vi "update FPS slider.vi"(8 "error in (no error)":errorcluster, 11 "Thorcam in":refnum<class "Thorcam.lvclass">) -> (0 "error out":errorcluster, 3 "Thorcam out":refnum<class "Thorcam.lvclass">)   [LabVIEW 2012, in "Thorcam.lvclass"]
uses:
  Thorcam.lvclass
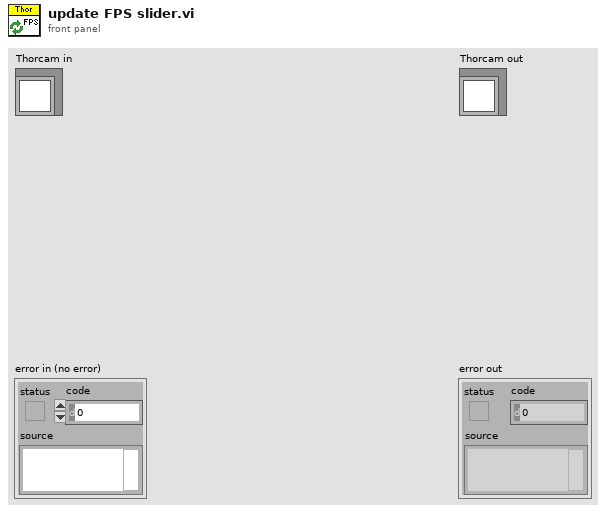
[diagram p1: front panel]
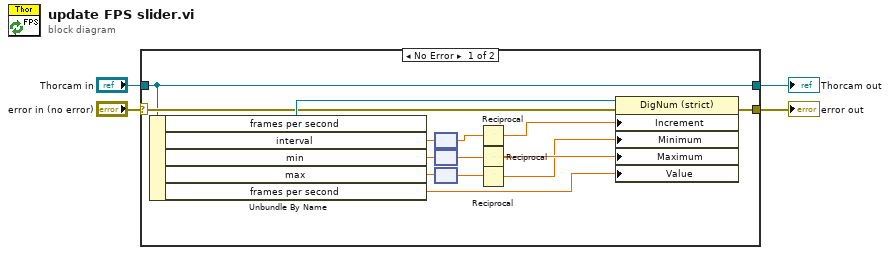
[diagram p0: block diagram]
diagram:
  n1 = case shown="No Error" "error in (no error)" {
    selector: "error in (no error)" -> [w16 w20]
    tunnel: [w17 w20] -> w3
    tunnel: [w15 w19] -> w1
    tunnel: "Thorcam in" -> [w15 w19]
    frame No Error {
      n2 = Unbundle By Name(w15) -> ("frames per second"=w18:refnum<vi>, "interval"=w6:dbl[unit], "min"=w12:dbl[unit], "max"=w11:dbl[unit], "frames per second"=w5:dbl)
      n3 = node(w6) -> (w7:dbl)
      n4 = node(w12) -> (w14:dbl)
      n5 = node(w11) -> (w13:dbl)
      n6 = Reciprocal(x=w7) -> (1/x=w8:dbl)
      n7 = Reciprocal(x=w14) -> (1/x=w10:dbl)
      n8 = Reciprocal(x=w13) -> (1/x=w9:dbl)
      n9 = property class="DigNum (strict)"(reference=w18, error in=w16, "Increment"=w8, "Minimum"=w9, "Maximum"=w10, "Value"=w5) -> (error out=w17:errorcluster)  [unwired: 1 out]
    }
    frame Error {
    }
  }
  "error out" <- w3
  "Thorcam out" <- w1
